vi "duplicate channel.vi"(8 "number of available channels":u16, 10 "Sensor Array":T1, 11 "Numeric":u32) -> (2 "Sensor Array out":T1, 3 "IndexVals":u32)   [LabVIEW 2012]
uses:
  DAQ configuration/Sensor array.ctl
  DAQ configuration/channel identifier.ctl
  global scale array.vi
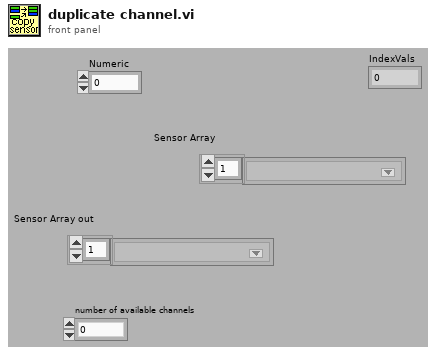
[diagram p1: front panel]
types:
  T1 = typedef "Sensor array.ctl" = T2[]
  T2 = typedef "channel identifier.ctl" = u16
  T3 = typedef "calib array.ctl" = T4[]
  T4 = typedef "conversion.ctl" = cluster{"conversion matrix":sgl[][], "units":string, "name":string, "scale type":T5, "offset (volts)":dbl, "second channel":i8, "correspondence table":T6, "offset (physical units)":dbl, "pH scale":T7, "D.O.":T8}
  T5 = typedef "scale type.ctl" = enum16{"Volts", "Polynomial", "Correspondence Table", "pH", "Dissolved Oxygen", "Quadratic"}
  T6 = typedef "correspondence table.ctl" = cluster{"physical units":dbl, "volts":dbl}[]
  T7 = typedef "pH scale.ctl" = cluster{"Buffers":cluster{"Buffer":dbl, "Calibrated":bool, "V/T":dbl}[], "Temperature":dbl}
  T8 = typedef "DO scale.ctl" = cluster{"Temperature":dbl, "K":dbl, "barometric pressure":dbl}
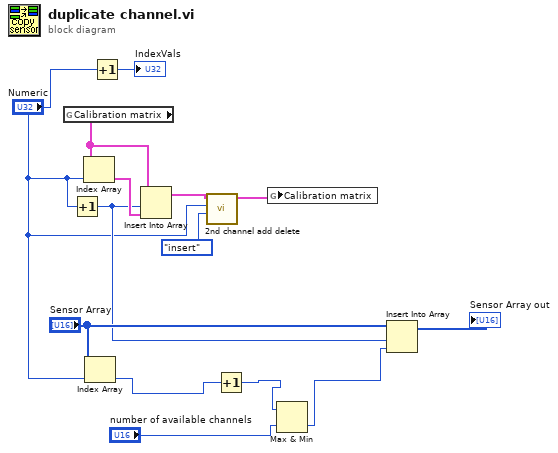
[diagram p0: block diagram]
diagram:
  n1 = global read "global scale array.vi" "Calibration matrix"() -> (w12:T3)
  n2 = Increment(x="Numeric") -> (x+1=w10:u32)
  n3 = Index Array(array=w12, index="Numeric") -> (element=w11:T4)
  n4 = Index Array(array="Sensor Array", index="Numeric") -> (element=w4:T2)
  n5 = Increment(x="Numeric") -> (x+1=→"IndexVals":u32)
  n6 = Insert Into Array(array=w12, index=w10, new element=w11) -> (w9:T3)
  n7 = call "2nd channel add delete.vi"("action"=enum16{"delete", "insert"}."insert", "Index"="Numeric", "Calibration array"=w9) -> ("Calibration array out"=w8:T3)  [unwired: 8 in]
  n8 = Increment(x=w4) -> (x+1=w2:T2)
  n9 = global write "global scale array.vi" "Calibration matrix"(w8) -> ()
  n10 = Max & Min(x=w2, y="number of available channels") -> (min(x,y)=w1:T2)  [unwired: 1 out]
  n11 = Insert Into Array(array="Sensor Array", index=w10, new element=w1) -> (→"Sensor Array out":T1)
